vi "SMO.BasicByRef.SetData.vi"(8 "error in (no error)":errorcluster, 10 "Value":T1, 11 "SMO.BasicByRef":refnum<class "SMO.BasicByRef.lvclass">) -> (0 "error out":errorcluster, 3 "SMO.BasicByRef out":refnum<class "SMO.BasicByRef.lvclass">)   [LabVIEW 2019, in "SMO.BasicByRef.lvclass"]
doc: "---------------------------------------------------------------\nJKI State Machine Objects™\nhttp://jki.net/state-machine-objects/\nCopyright (C) 2005-2015, JKI <info@jki.net>\nALL RIGHTS RESERVEDJKI State Machine Objects (SMO) 1.0.0.5\nJKI - JKI\nCopyright (c) 2016, JKI"
uses:
  SMO.BasicByRef.lvclass
  Typedefs/Value.ctl
  SMO.BasicByRef.lvclass/SMO.BasicByRef.ctl
  Typedefs/ValueChanged--EventData--Cluster.ctl
panel:
  # "For instructions on how to use the JKI State Machine Objects, examples and video tutorials, visit:\nhttp://jki.net/state-machine-objects/\n\nJKI State Machine Objects™\nhttp://jki.net/state-machine-objects/\nCopyright (C) 2005-2015, JKI <info@jki.net>\nALL RIGHTS RESERVED"
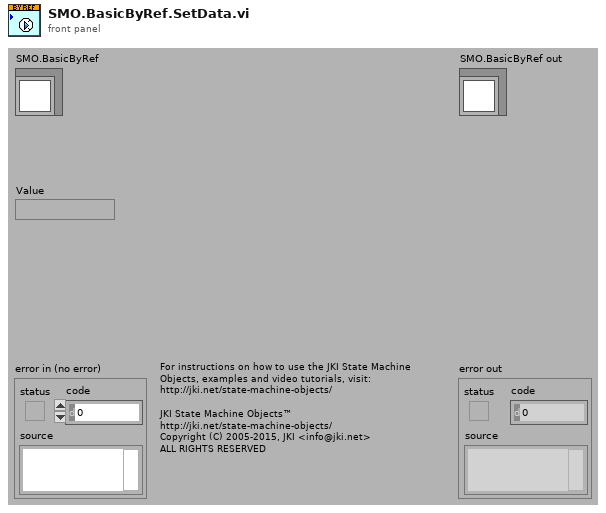
[diagram p1: front panel]
types:
  T1 = typedef "SMO.BasicByRef.lvclass/Value.ctl" = string
  T2 = typedef "SMO.BasicByRef.lvclass/ValueChanged--EventData--Cluster.ctl" = cluster{"New Value":string}
  T3 = typedef "SMO.BasicByRef.lvclass/PrivateData--Ref.ctl" = refnum<data-value>
  T4 = typedef "SMO.BasicByRef.lvclass/PrivateData--Cluster.ctl" = cluster{"Public Events":T5, "Protected Events":T6, "Private Events":T7, "Value":T1}
  T5 = typedef "SMO.BasicByRef.lvclass/PublicEvents--Cluster.ctl" = cluster{"Value Changed":refnum<user-event>}
  T6 = typedef "SMO.BasicByRef.lvclass/ProtectedEvents--Cluster.ctl" = cluster{"placeholder":refnum<user-event>}
  T7 = typedef "SMO.BasicByRef.lvclass/PrivateEvents--Cluster.ctl" = cluster{"New Value":refnum<user-event>}
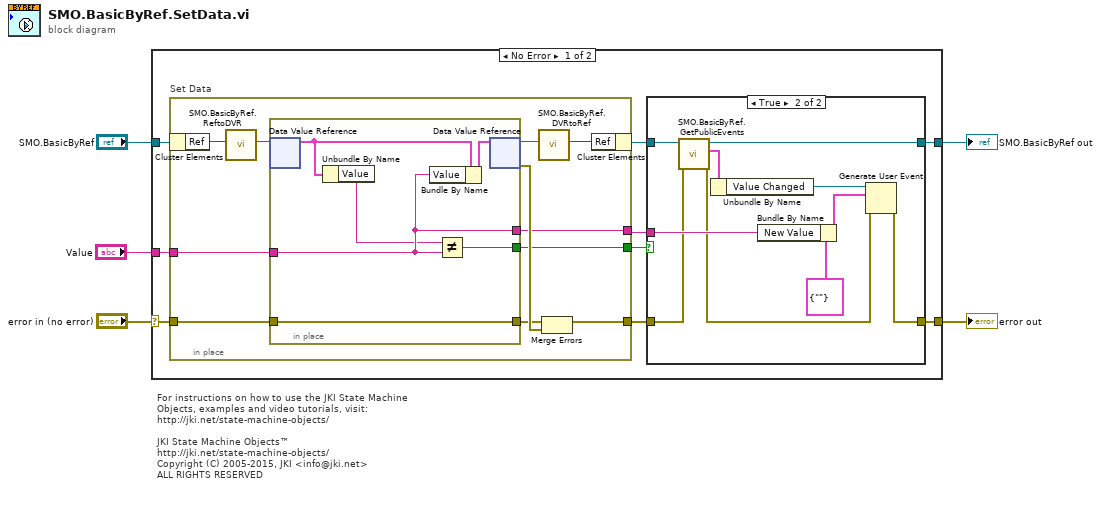
[diagram p0: block diagram]
diagram:
  # "For instructions on how to use the JKI State Machine Objects, examples and video tutorials, visit:\nhttp://jki.net/state-machine-objects/\n\nJKI State Machine Objects™\nhttp://jki.net/state-machine-objects/\nCopyright (C) 2005-2015, JKI <info@jki.net>\nALL RIGHTS RESERVED"
  n1 = case shown="No Error" "error in (no error)" {
    selector: "error in (no error)" -> [w12 w44]
    tunnel: "SMO.BasicByRef" -> [w13 w45]
    tunnel: [w10 w44] -> w4
    tunnel: [w8 w45] -> w3
    tunnel: "Value" -> [w14 _]
    frame No Error {
      n2 = in-place "Set Data" {
        in-place-border: w12 -> [w37]
        in-place-border: [w34] -> w7
        in-place-border: w14 -> [w33]
        in-place-border: [w32] -> w11
        in-place-border: [w27] -> w6
        n3 = in-place-cluster #1(w13) -> ("Ref"=w31:u32)
        n4 = call "SMO.BasicByRef.ReftoDVR.vi"("Ref"=w31) -> ("Ref"=w30:T3)  [unwired: 10 in]
        n5 = in-place {
          in-place-border: w37 -> [w43]
          in-place-border: [w43] -> w35
          in-place-border: w33 -> [w40]
          in-place-border: [w40] -> w32
          in-place-border: [w38] -> w27
          n6 = in-place-dvr #2(w30) -> (w41:T4)  [unwired: 1 out]
          n7 = Unbundle By Name(w41) -> ("Value"=w39:T1)
          n8 = Bundle By Name(cluster=w41, "Value"=w40) -> (w42:T4)
          n9 = Not Equal?(x=w39, y=w40) -> (x != y?=w38:bool)
          n10 = in-place-dvr #2(w42) -> (w29:T3, w36:errorcluster)
        }
        n11 = call "SMO.BasicByRef.DVRtoRef.vi"("Ref"=w29) -> ("Ref"=w28:u32)  [unwired: 10 in]
        n12 = Merge Errors(w35, w36) -> (w34:errorcluster)
        n13 = in-place-cluster #1("Ref"=w28) -> (w9:refnum<class "SMO.BasicByRef.lvclass">)
      }
      n14 = case shown="True" w6 {
        tunnel: w11 -> [_ w23]
        tunnel: [w15 w22] -> w10
        tunnel: w9 -> [w16 w21]
        tunnel: [w16 w20] -> w8
        tunnel: w7 -> [w15 w18]
        frame False {
        }
        frame True {
          n15 = call "SMO.BasicByRef.GetPublicEvents.vi"("error in (no error)"=w18, "SMO.BasicByRef"=w21) -> ("error out"=w17:errorcluster, "SMO.BasicByRef Public Events"=w19:T5, "SMO.BasicByRef out"=w20:refnum<class "SMO.BasicByRef.lvclass">)  [unwired: 7 in]
          n16 = Unbundle By Name(w19) -> ("Value Changed"=w26:refnum<user-event>)
          n17 = Bundle By Name(cluster=T2 {"New Value"=""} ("event data"), "New Value"=w23) -> (w24:T2)
          n18 = Generate User Event(user event=w26, event data cluster=w24, error in=w17) -> (error out=w22:errorcluster)  [unwired: 1 in, 1 out]
        }
      }
    }
    frame Error {
    }
  }
  "error out" <- w4
  "SMO.BasicByRef out" <- w3
